vi "Normalize2DGaussianParameters.vi"(1 "best fit parameters IN":dbl[](array[numeric])) -> (0 "best fit parameters OUT":dbl[](array[numeric]))   [LabVIEW 2009]
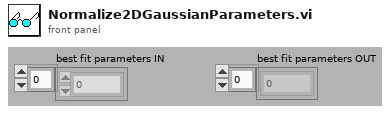
[diagram p1: front panel]
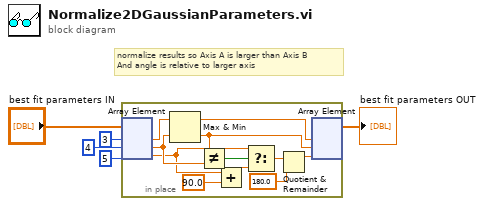
[diagram p0: block diagram]
diagram:
  # "normalize results so Axis A is larger than Axis B\nAnd angle is relative to larger axis"
  n1 = in-place {
    n2 = in-place-array #1("best fit parameters IN", 3, 4, 5) -> (w15:dbl, w12:dbl, w8:dbl)
    n3 = Max & Min(x=w15, y=w12) -> (max(x,y)=w14:dbl, min(x,y)=w13:dbl)
    n4 = Not Equal?(x=w13, y=w12) -> (x != y?=w9:bool)
    n5 = Add(x=w8, y=90.0) -> (x+y=w7:dbl)
    n6 = Select(t=w8, s=w9, f=w7) -> (s? t:f=w10:dbl)
    n7 = Quotient & Remainder(x=w10, y=180.0) -> (x-y*floor(x/y)=w16:dbl)  [unwired: 1 out]
    n8 = in-place-array #1(w14, w13, w16) -> (→"best fit parameters OUT":dbl[])  [unwired: 3 out]
  }
